vi "Coerce Sample Rate.vi"(9 "Sample Rate:":dbl, 10 "Maximum":dbl, 11 "Sample Rate Unit":enum16{"Hz", "kHz", "MHz"}(ring)) -> (2 "Coercion needed?":bool, 3 "Actual Sample Rate (s)":dbl)   [LabVIEW 2021]
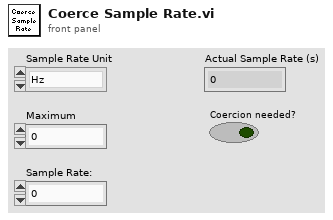
[diagram p1: front panel]
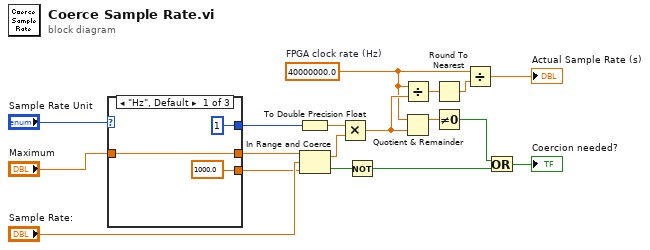
[diagram p0: block diagram]
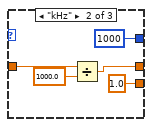
[diagram p2: hidden frame]
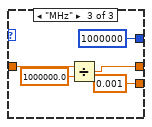
[diagram p3: hidden frame]
diagram:
  w1 = 40000000.0  # FPGA clock rate (Hz)
  n1 = case shown="\"Hz\", Default" "Sample Rate Unit" {
    tunnel: [1 1000 1000000] -> w14
    tunnel: [w19 w22 w27] -> w13
    tunnel: [1000.0 ("Data Entry Limits:Minimum") 1.0 ("Data Entry Limits:Minimum") 0.001 ("Data Entry Limits:Minimum")] -> w12
    tunnel: "Maximum" -> [w19 w24 w29]
    frame "Hz", Default {
    }
    frame "kHz" {
      n2 = Divide(x=w24, y=1000.0) -> (x/y=w22:dbl)
    }
    frame "MHz" {
      n3 = Divide(x=w29, y=1000000.0) -> (x/y=w27:dbl)
    }
  }
  n4 = To Double Precision Float(number=w14) -> (double precision float=w10:dbl)
  n5 = In Range and Coerce(upper limit=w13, x="Sample Rate:", lower limit=w12) -> (coerced(x)=w11:dbl, In Range?=w8:bool)
  n6 = Multiply(x=w10, y=w11) -> (x*y=w6:dbl)
  n7 = Not(x=w8) -> (.not. x?=w7:bool)
  n8 = Divide(x=w1, y=w6) -> (x/y=w9:dbl)
  n9 = Quotient & Remainder(x=w1, y=w6) -> (x-y*floor(x/y)=w5:dbl)  [unwired: 1 out]
  n10 = Round To Nearest(number=w9) -> (nearest integer value=w2:dbl)
  n11 = Not Equal To 0?(x=w5) -> (x != 0?=w3:bool)
  n12 = Divide(x=w1, y=w2) -> (x/y=→"Actual Sample Rate (s)":dbl)
  n13 = Or(x=w3, y=w7) -> (x .or. y?=→"Coercion needed?":bool)
